vi "Fieldbus_Write_message.vi"(8 "error in":errorcluster, 9 "Data":i32, 11 "Message":string) -> (0 "error output":errorcluster, 3 "Write":T1)   [LabVIEW 2021]
panel:
  out "Message Output":T1
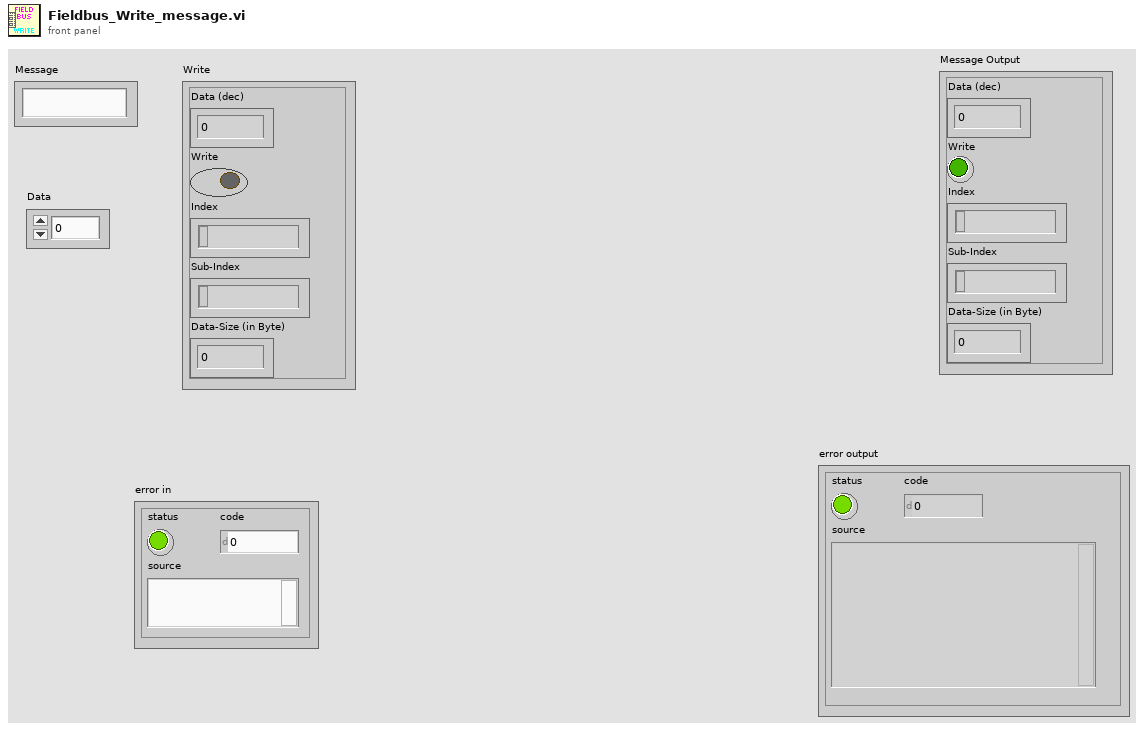
[diagram p1: front panel]
types:
  T1 = cluster{"Data (dec)":i32, "Write":bool, "Index":string, "Sub-Index":string, "Data-Size (in Byte)":u8}
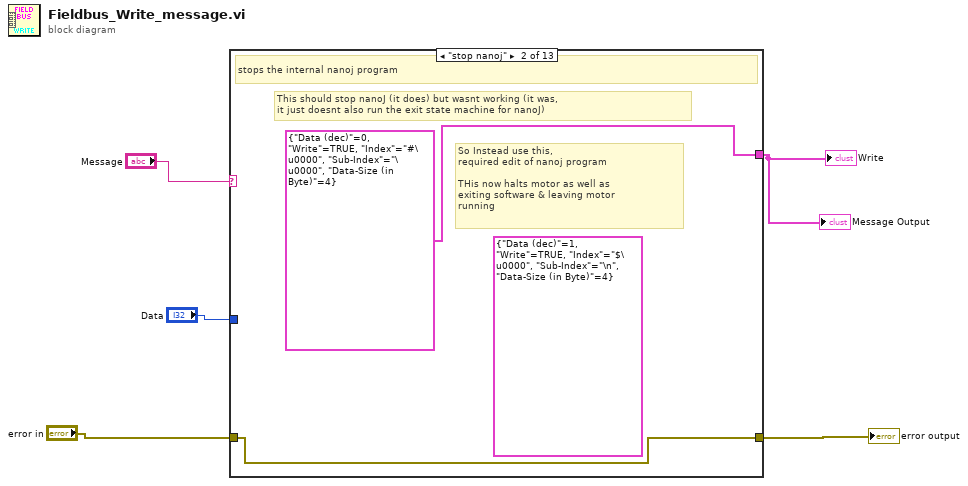
[diagram p0: block diagram]
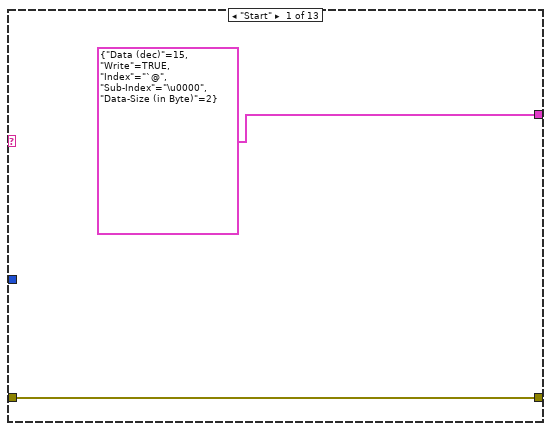
[diagram p2: hidden frame]
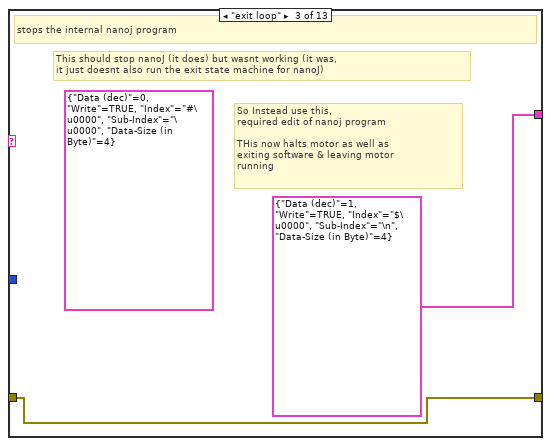
[diagram p3: hidden frame]
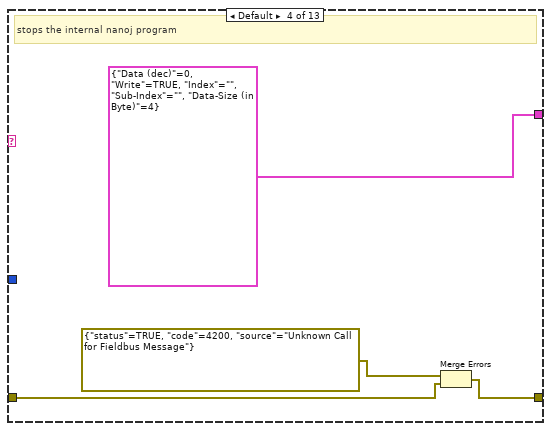
[diagram p4: hidden frame]
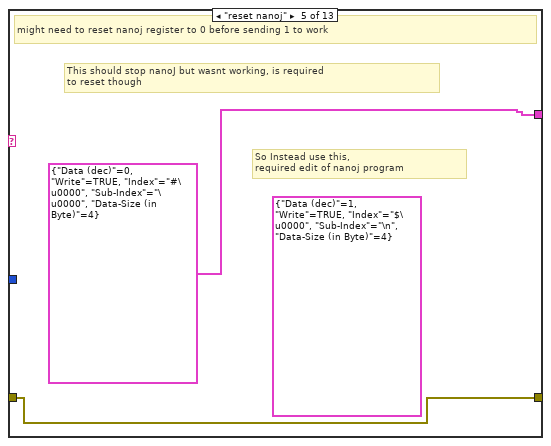
[diagram p5: hidden frame]
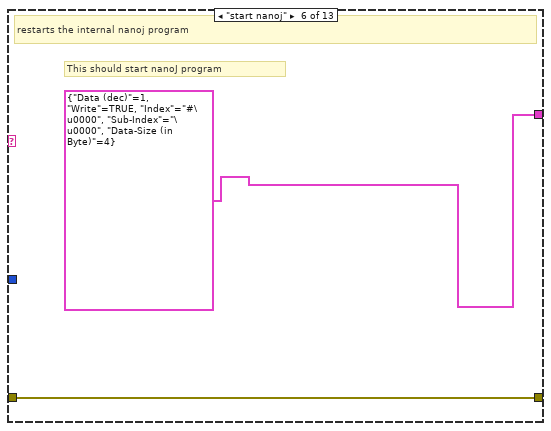
[diagram p6: hidden frame]
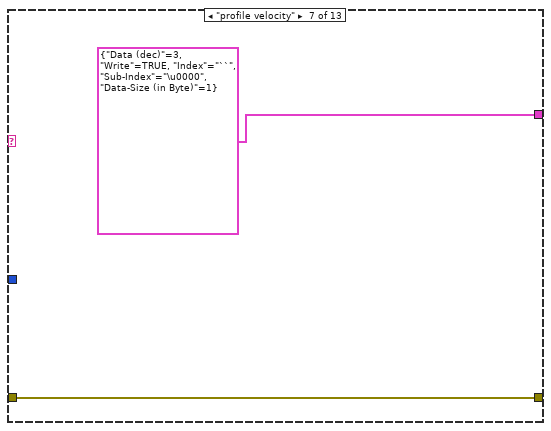
[diagram p7: hidden frame]
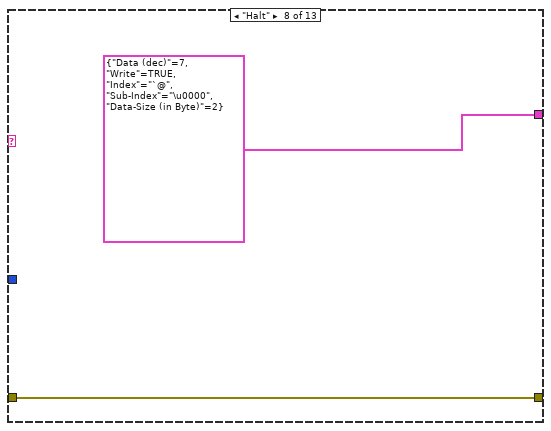
[diagram p8: hidden frame]
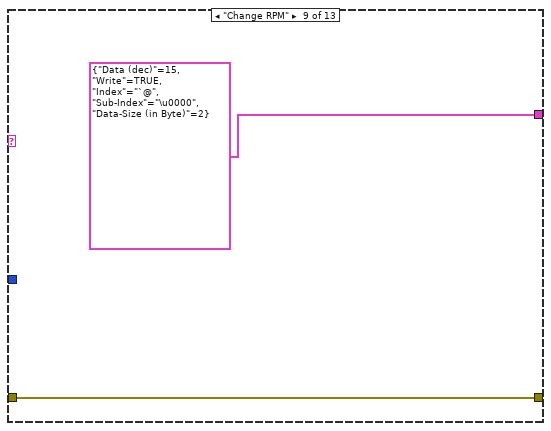
[diagram p9: hidden frame]
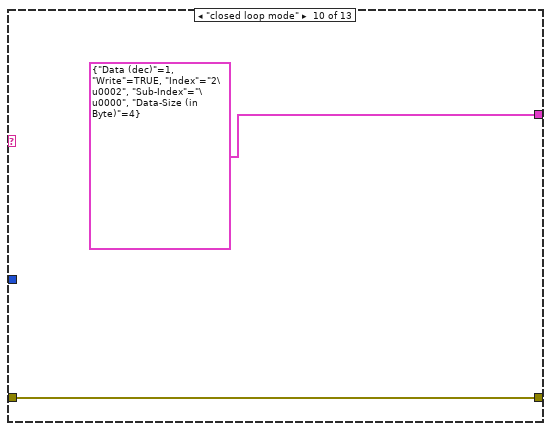
[diagram p10: hidden frame]
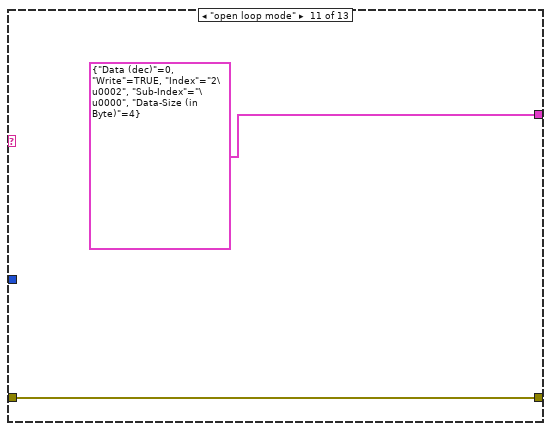
[diagram p11: hidden frame]
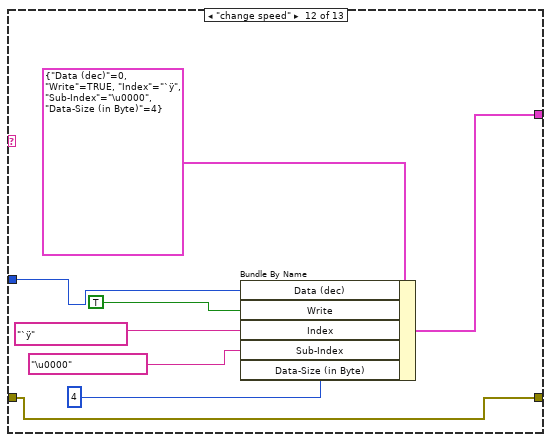
[diagram p12: hidden frame]
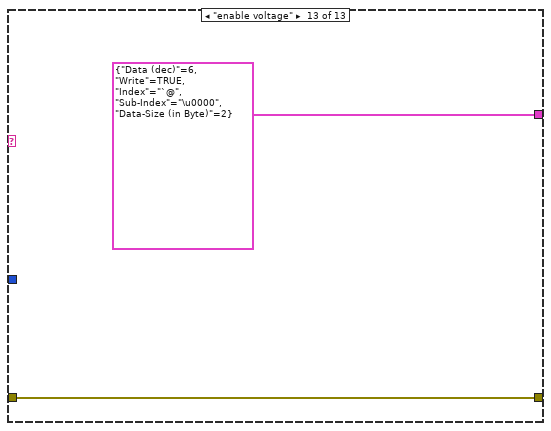
[diagram p13: hidden frame]
diagram:
  n1 = case shown="\"stop nanoj\"" "Message" {
    tunnel: [T1 {"Data (dec)"=15, "Write"=TRUE, "Index"="`@", "Sub-Index"="\u0000", "Data-Size (in Byte)"=2} ("Write") T1 {"Data (dec)"=0, "Write"=TRUE, "Index"="#\u0000", "Sub-Index"="\u0000", "Data-Size (in Byte)"=4} ("Write") T1 {"Data (dec)"=1, "Write"=TRUE, "Index"="$\u0000", "Sub-Index"="\n", "Data-Size (in Byte)"=4} ("Write") T1 {"Data (dec)"=0, "Write"=TRUE, "Index"="", "Sub-Index"="", "Data-Size (in Byte)"=4} ("Write") T1 {"Data (dec)"=0, "Write"=TRUE, "Index"="#\u0000", "Sub-Index"="\u0000", "Data-Size (in Byte)"=4} ("Write") T1 {"Data (dec)"=1, "Write"=TRUE, "Index"="#\u0000", "Sub-Index"="\u0000", "Data-Size (in Byte)"=4} ("Write") T1 {"Data (dec)"=3, "Write"=TRUE, "Index"="``", "Sub-Index"="\u0000", "Data-Size (in Byte)"=1} ("Write") T1 {"Data (dec)"=7, "Write"=TRUE, "Index"="`@", "Sub-Index"="\u0000", "Data-Size (in Byte)"=2} ("Write") T1 {"Data (dec)"=15, "Write"=TRUE, "Index"="`@", "Sub-Index"="\u0000", "Data-Size (in Byte)"=2} ("Write") T1 {"Data (dec)"=1, "Write"=TRUE, "Index"="2\u0002", "Sub-Index"="\u0000", "Data-Size (in Byte)"=4} ("Write") T1 {"Data (dec)"=0, "Write"=TRUE, "Index"="2\u0002", "Sub-Index"="\u0000", "Data-Size (in Byte)"=4} ("Write") w36 T1 {"Data (dec)"=6, "Write"=TRUE, "Index"="`@", "Sub-Index"="\u0000", "Data-Size (in Byte)"=2} ("Write")] -> w5
    tunnel: "Data" -> [_ _ _ _ _ _ _ _ _ _ _ w35 _]
    tunnel: [w6 w9 w10 w13 w16 w18 w20 w22 w24 w26 w28 w30 w38] -> w2
    tunnel: "error in" -> [w6 w9 w10 w12 w16 w18 w20 w22 w24 w26 w28 w30 w38]
    frame "Start" {
    }
    frame "stop nanoj" {
      (unwired) T1 {"Data (dec)"=1, "Write"=TRUE, "Index"="$\u0000", "Sub-Index"="\n", "Data-Size (in Byte)"=4} ("Write")
      # "So Instead use this,\nrequired edit of nanoj program\n\nTHis now halts motor as well as\nexiting software & leaving motor\nrunning"
      # "This should stop nanoJ (it does) but wasnt working (it was,\nit just doesnt also run the exit state machine for nanoJ)"
      # "stops the internal nanoj program"
    }
    frame "exit loop" {
      (unwired) T1 {"Data (dec)"=0, "Write"=TRUE, "Index"="#\u0000", "Sub-Index"="\u0000", "Data-Size (in Byte)"=4} ("Write")
      # "So Instead use this,\nrequired edit of nanoj program\n\nTHis now halts motor as well as\nexiting software & leaving motor\nrunning"
      # "This should stop nanoJ (it does) but wasnt working (it was,\nit just doesnt also run the exit state machine for nanoJ)"
      # "stops the internal nanoj program"
    }
    frame Default {
      # "stops the internal nanoj program"
      n2 = Merge Errors(errorcluster {"status"=TRUE, "code"=4200, "source"="Unknown Call for Fieldbus Message"} ("error constant"), w12) -> (w13:errorcluster)
    }
    frame "reset nanoj" {
      (unwired) T1 {"Data (dec)"=1, "Write"=TRUE, "Index"="$\u0000", "Sub-Index"="\n", "Data-Size (in Byte)"=4} ("Write")
      # "So Instead use this,\nrequired edit of nanoj program"
      # "This should stop nanoJ but wasnt working, is required\nto reset though"
      # "might need to reset nanoj register to 0 before sending 1 to work"
    }
    frame "start nanoj" {
      # "This should start nanoJ program"
      # "restarts the internal nanoj program"
    }
    frame "profile velocity" {
    }
    frame "Halt" {
    }
    frame "Change RPM" {
    }
    frame "closed loop mode" {
    }
    frame "open loop mode" {
    }
    frame "change speed" {
      n3 = Bundle By Name(cluster=T1 {"Data (dec)"=0, "Write"=TRUE, "Index"="`ÿ", "Sub-Index"="\u0000", "Data-Size (in Byte)"=4} ("Write"), "Data (dec)"=w35, "Write"=TRUE, "Index"="`ÿ", "Sub-Index"="\u0000", "Data-Size (in Byte)"=u8 4) -> (w36:T1)
    }
    frame "enable voltage" {
    }
  }
  "Write" <- w5
  "Message Output" <- w5
  "error output" <- w2
